vi "VI Tree - lvdata__ogtk.vi"() -> ()   [LabVIEW 2009]
uses:
  Type Descriptor Enumeration__ogtk.ctl
  Type Descriptor Header__ogtk.ctl
  Refnum Code__ogtk.ctl
  Base Units__ogtk.ctl
  Physical Units__ogtk.ctl
  Type Descriptor__ogtk.ctl
panel:
  in  "Type Descriptor":T1
  in  "Physical Units":T2
  in  "Base Units":T3
  in  "Refnum Code":T4
  out "Type Descriptor Header":T5 {"type" format="%.0x"}
  in  "Type Descriptor Enumeration":T6 format="%.0x"
  # "[OpenG VI Tags] ***Do Not Remove***"
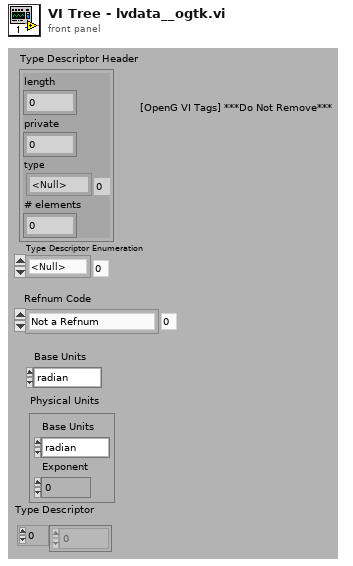
[diagram p1: front panel]
types:
  T1 = typedef "Type Descriptor__ogtk.ctl" = i16[]
  T2 = typedef "Physical Units__ogtk.ctl" = cluster{"Base Units":enum16{"radian", "steradian", "second", "meter", "kilogram", "ampere", "kelvin", "mole", "candela"}, "Exponent":i16}
  T3 = typedef "Base Units__ogtk.ctl" = enum16{"radian", "steradian", "second", "meter", "kilogram", "ampere", "kelvin", "mole", "candela"}
  T4 = typedef "Refnum Code__ogtk.ctl" = enum16{"Not a Refnum", "Datalog File", "Byte Stream File", "0x03", "Occurence", "TCP", "0x06", "ActiveX", "Generic VI Server Class", "Menu", "0x0A", "IMAQ Session", "0x0C", "0x0D", "VISA", "IVI", "UDP"}
  T5 = typedef "Type Descriptor Header__ogtk.ctl" = cluster{"length":u16, "private":u8, "type":T6, "# elements":u16}
  T6 = typedef "Type Descriptor Enumeration__ogtk.ctl" = enum8{"<Null>", "I8", "I16", "I32", "I64", "U8", "U16", "U32", "U64", "SGL", "DBL", "EXT", "CSG", "CDB", "CXT", "0x0F", "0x10", "0x11", "0x12", "0x13", "0x14", "Enum U8", "Enum U16", "Enum U32", "Enum U64", "SGL PQ", "DBL PQ", "EXT PQ", "CSG PQ", "CDB PQ", "CXT PQ", "0x1F", "0x20", "Boolean", "0x22", "0x23", "0x24", "0x25", "0x26", "0x27", "0x28", "0x29", "0x2A", "0x2B", "0x2C", "0x2D", "0x2E", "0x2F", "String", "0x31", "Path", "Pict", "0x34", "0x35", "0x36", "DAQ", "0x38", "0x39", "0x3A", "0x3B", "0x3C", "0x3D", "0x3E", "0x3F", "Array", "0x41", "0x42", "0x43", "0x44", "0x45", "0x46", "0x47", "0x48", "0x49", "0x4A", "0x4B", "0x4C", "0x4D", "0x4E", "0x4F", "Cluster", "0x51", "0x52", "Variant", "Waveform", "0x55", "0x56", "0x57", "0x58", "0x59", "0x5A", "0x5B", "0x5C", "0x5D", "0x5E", "0x5F", "0x60", "0x61", "0x62", "0x63", "0x64", "0x65", "0x66", "0x67", "0x68", "0x69", "0x6A", "0x6B", "0x6C", "0x6D", "0x6E", "0x6F", "Refnum"}
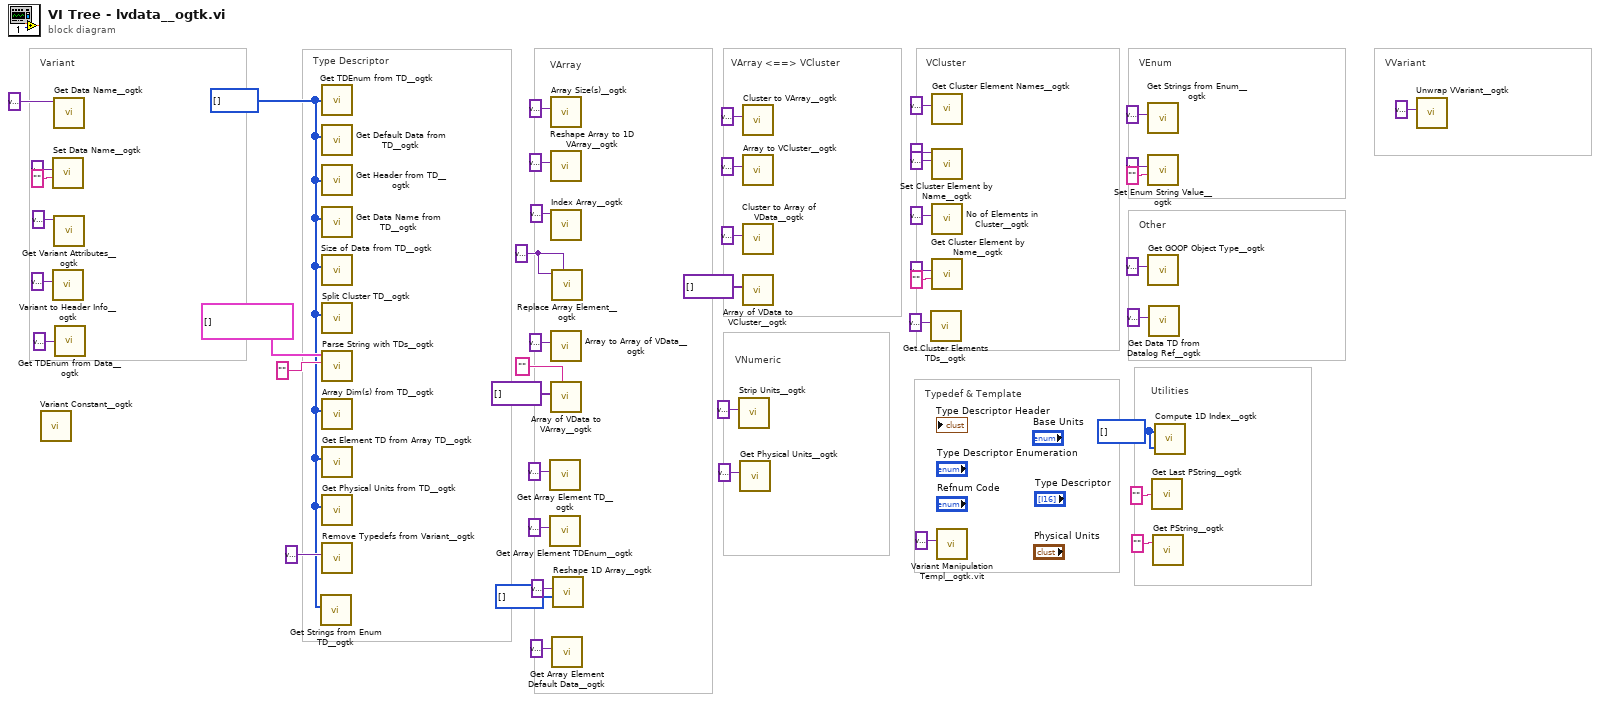
[diagram p0: block diagram]
diagram:
  w12 = variant ("New Element")
  w32 = u32[] [] ("Indices")
  w6 = T1 [] ("Type Descriptor")
  # "VVariant"
  # "VNumeric"
  # "Other"
  # "Type Descriptor"
  # "Typedef & Template"
  # "Variant"
  # "Utilities"
  # "VEnum"
  # "VArray <==> VCluster"
  # "VCluster"
  # "VArray"
  n1 = call "Variant Constant__ogtk.vi"() -> ()  [unwired: 1 in]
  n2 = call "Set Data Name__ogtk.vi"("Data Name"="", "Data"=variant) -> ()  [unwired: 8 in, 2 out]
  n3 = call "Variant to Header Info__ogtk.vi"("Variant"=variant) -> ()  [unwired: 3 in, 3 out]
  n4 = call "Get Data Name__ogtk.vi"("Data"=variant) -> ()  [unwired: 8 in, 3 out]
  n5 = call "Get Variant Attributes__ogtk.vi"("Variant"=variant) -> ()  [unwired: 3 in, 4 out]
  n6 = call "Get TDEnum from Data__ogtk.vi"("Data"=variant) -> ()  [unwired: 4 in, 1 out]
  n7 = call "Get Strings from Enum TD__ogtk.vi"("Type Descriptor"=w6) -> ()  [unwired: 8 in, 3 out]
  n8 = call "Get TDEnum from TD__ogtk.vi"("Type Descriptor"=w6) -> ()  [unwired: 4 in, 1 out]
  n9 = call "Get Default Data from TD__ogtk.vi"("Type Descriptor"=w6) -> ()  [unwired: 9 in, 2 out]
  n10 = call "Get Header from TD__ogtk.vi"("Type Descriptor"=w6) -> ()  [unwired: 1 out]
  n11 = call "Get Data Name from TD__ogtk.vi"("Type Descriptor"=w6) -> ()  [unwired: 9 in, 2 out]
  n12 = call "Size of Data from TD__ogtk.vi"("Type Descriptor"=w6) -> ()  [unwired: 9 in, 2 out]
  n13 = call "Split Cluster TD__ogtk.vi"("Type Descriptor"=w6) -> ()  [unwired: 9 in, 2 out]
  n14 = call "Parse String with TDs__ogtk.vi"("Data string"="", "Type Descriptors"=cluster{"Type Descriptor":T1}[] []) -> ()  [unwired: 7 in, 3 out]
  n15 = call "Array Dim(s) from TD__ogtk.vi"("Array Type Descriptor"=w6) -> ()  [unwired: 9 in, 2 out]
  n16 = call "Get Element TD from Array TD__ogtk.vi"("Array Type Descriptor"=w6) -> ()  [unwired: 9 in, 2 out]
  n17 = call "Get Physical Units from TD__ogtk.vi"("Float or Array Type Descriptor"=w6) -> ()  [unwired: 9 in, 2 out]
  n18 = call "Remove Typedefs from Variant__ogtk.vi"("Variant with typedefs"=variant) -> ()  [unwired: 9 in, 2 out]
  n19 = call "Get Array Element TD__ogtk.vi"("Array"=variant) -> ()  [unwired: 9 in, 2 out]
  n20 = call "Get Array Element TDEnum__ogtk.vi"("Array"=variant) -> ()  [unwired: 9 in, 2 out]
  n21 = call "Array Size(s)__ogtk.vi"("Array"=variant) -> ()  [unwired: 8 in, 3 out]
  n22 = call "Reshape Array to 1D VArray__ogtk.vi"("MultiD Array"=variant) -> ()  [unwired: 8 in, 3 out]
  n23 = call "Index Array__ogtk.vi"("MultiD Array"=variant) -> ()  [unwired: 9 in, 2 out]
  n24 = call "Array to Array of VData__ogtk.vi"("MultiD Array"=variant) -> ()  [unwired: 9 in, 2 out]
  n25 = call "Array of VData to VArray__ogtk.vi"("Array Name"="", "1D Array of VData"=variant[] []) -> ()  [unwired: 8 in, 2 out]
  n26 = call "Replace Array Element__ogtk.vi"("New Element"=w12, "MultiD Array"=w12) -> ()  [unwired: 8 in, 2 out]
  n27 = call "Get Array Element Default Data__ogtk.vi"("Array"=variant) -> ()  [unwired: 9 in, 2 out]
  n28 = call "Reshape 1D Array__ogtk.vi"("Size(s)"=u32[] [], "1D Array"=variant) -> ()  [unwired: 8 in, 2 out]
  n29 = call "Strip Units__ogtk.vi"("Number or 1D array with units"=variant) -> ()  [unwired: 9 in, 2 out]
  n30 = call "Get Physical Units__ogtk.vi"("Float or Array of Floats"=variant) -> ()  [unwired: 9 in, 2 out]
  n31 = call "Cluster to VArray__ogtk.vi"("Cluster"=variant) -> ()  [unwired: 9 in, 2 out]
  n32 = call "Array to VCluster__ogtk.vi"("Array"=variant) -> ()  [unwired: 9 in, 2 out]
  n33 = call "Cluster to Array of VData__ogtk.vi"("Cluster"=variant) -> ()  [unwired: 9 in, 2 out]
  n34 = call "Array of VData to VCluster__ogtk.vi"("Array"=variant[] []) -> ()  [unwired: 9 in, 2 out]
  n35 = call "Get Cluster Elements TDs__ogtk.vi"("Cluster"=variant) -> ()  [unwired: 9 in, 2 out]
  n36 = call "Get Cluster Element Names__ogtk.vi"("Cluster"=variant) -> ()  [unwired: 9 in, 2 out]
  n37 = call "Set Cluster Element by Name__ogtk.vi"("New Element Value"=variant, "Cluster"=variant) -> ()  [unwired: 7 in, 3 out]
  n38 = call "No of Elements in Cluster__ogtk.vi"("Cluster"=variant) -> ()  [unwired: 9 in, 2 out]
  n39 = call "Get Cluster Element by Name__ogtk.vi"("Element Name"="", "Cluster"=variant) -> ()  [unwired: 7 in, 3 out]
  n40 = call "Variant Manipulation Templ__ogtk.vit"("Variant"=variant) -> ()  [unwired: 10 in, 1 out]
  n41 = call "Get Strings from Enum__ogtk.vi"("Enum"=variant) -> ()  [unwired: 7 in, 4 out]
  n42 = call "Set Enum String Value__ogtk.vi"("String Value"="", "Default Enum Value"=variant) -> ()  [unwired: 8 in, 2 out]
  n43 = call "Get GOOP Object Type__ogtk.vi"("GOOP Refnum"=variant) -> ()  [unwired: 9 in, 2 out]
  n44 = call "Get Data TD from Datalog Ref__ogtk.vi"("Datalog Refnum"=variant) -> ()  [unwired: 9 in, 2 out]
  n45 = call "Get Last PString__ogtk.vi"("String"="") -> ()  [unwired: 2 out]
  n46 = call "Get PString__ogtk.vi"("String"="") -> ()  [unwired: 1 in, 2 out]
  n47 = call "Compute 1D Index__ogtk.vi"("Size(s)"=w32, "Indices"=w32) -> ()  [unwired: 1 out]
  n48 = call "Unwrap VVariant__ogtk.vi"("VVariant"=variant) -> ()  [unwired: 9 in, 2 out]
